vi "To String.vi"(8 "error in (no error)":errorcluster, 11 "Boolean Array in":refnum<class "Boolean Array.lvclass">) -> (0 "error out":errorcluster, 2 "String":string)   [LabVIEW 2020, in "Data.lvlib" / "Boolean Array.lvclass"]
doc: "Convert 'Generic Data in' to a string."
uses:
  Boolean Array.lvclass
  Boolean Array.lvclass/Boolean Array.ctl
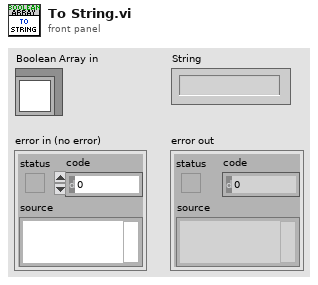
[diagram p1: front panel]
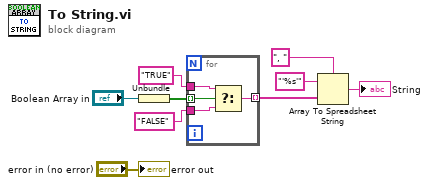
[diagram p0: block diagram]
diagram:
  n1 = Unbundle("Boolean Array in") -> (w4:bool[])
  n2 = for {
    tunnel: w4 -> [w13] mode=indexing
    tunnel: [w12] -> w3 mode=indexing
    tunnel: "TRUE" ("String 2") -> [w11]
    tunnel: "FALSE" ("f") -> [w10]
    n3 = Select(t=w11, s=w13, f=w10) -> (s? t:f=w12:string)
  }
  n4 = Array To Spreadsheet String(delimiter (Tab)=", ", array=w3, 3:"'%s'" ("format string")) -> (spreadsheet string=→"String":string)
  "error out" <- "error in (no error)"
